vi "SVT Human Vibration Weighting Filter (frequency).vi"   [LabVIEW 2017, in "SoundVib_HumanVibration.lvlib"]
doc: "Applies the selected human vibration weighting to FFT-based spectra. This VI weights each spectral bin according to the attenuation of the specified filter at the bin center frequency. This VI does not maintain state internally; you can use this VI in a loop to process multiple blocks. Wire data to the <B>spectrum</B> input to determine the polymorphic instance to use or manually select the instance."
uses:
  <vilib>/addons/Sound and Vibration/svt_Weighting/SoundVib_HumanVibration.lvlib
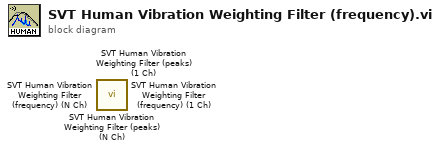
[diagram p0: block diagram]
diagram:
  n1 = call <vilib>:"SVT Human Vibration Weighting Filter (peaks) (N Ch).vi"() -> ()  [unwired: 16 in, 4 out]
  n2 = call <vilib>:"SVT Human Vibration Weighting Filter (peaks) (1 Ch).vi"() -> ()  [unwired: 16 in, 4 out]
  n3 = call <vilib>:"SVT Human Vibration Weighting Filter (frequency) (N Ch).vi"() -> ()  [unwired: 16 in, 4 out]
  n4 = call <vilib>:"SVT Human Vibration Weighting Filter (frequency) (1 Ch).vi"() -> ()  [unwired: 16 in, 4 out]
